vi "Find Candidates.vi"(0 "Target Heading":i16, 1 "Number of Valleys":i16, 2 "START":i16[](array[numeric]), 3 "STOP":i16[](array[numeric]), 5 "Expansion delta":i16) -> (4 "Valley index":i16, 6 "Candidate Direction":i16[](array[numeric]), 7 "Valley Width":i16[](array[numeric]), 8 "Target Bonus":i16[](array[numeric]))   [LabVIEW 2009]
panel:
  out "Target Valley Width":i16
  out "Target Flag":i16
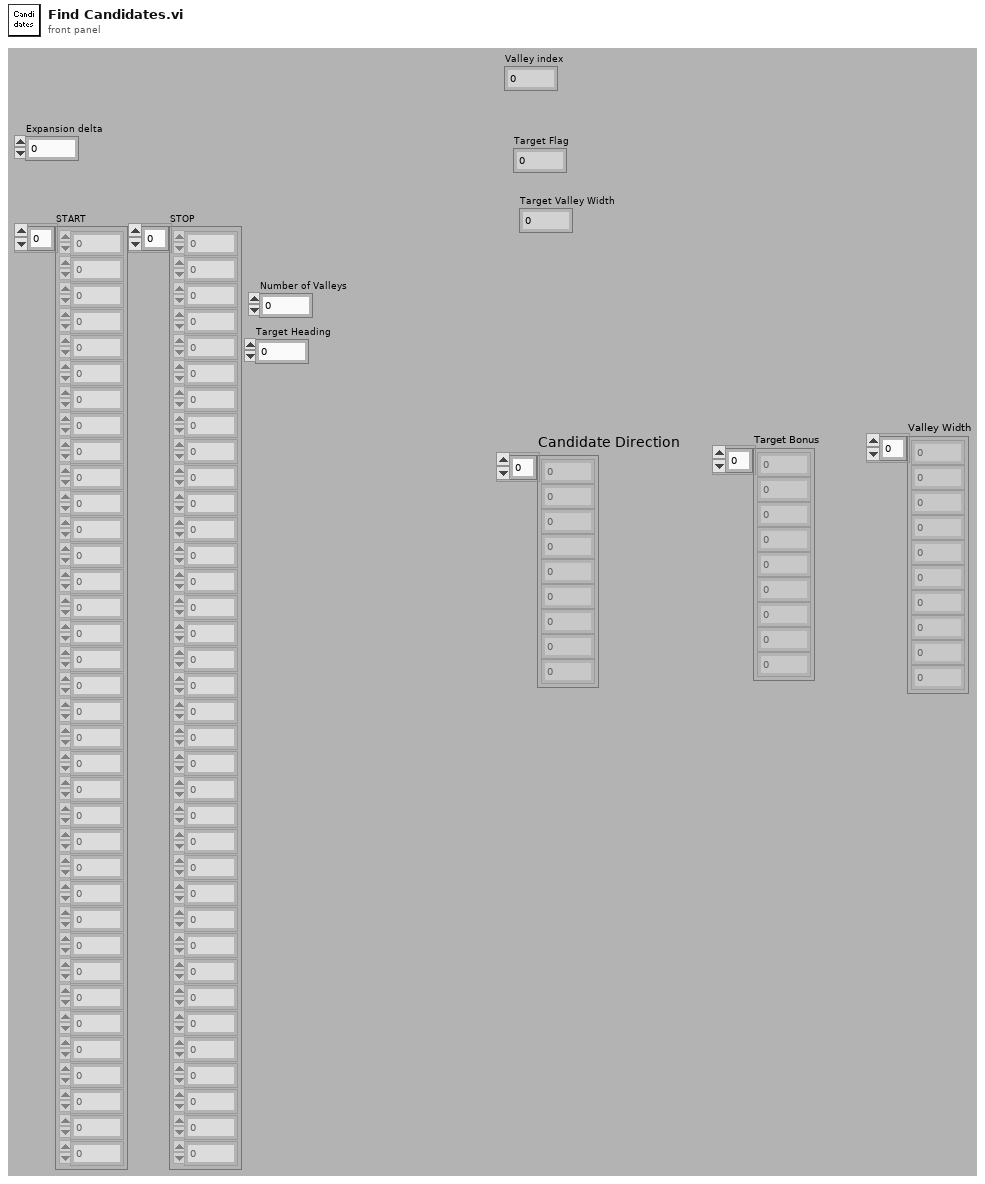
[diagram p1: front panel]
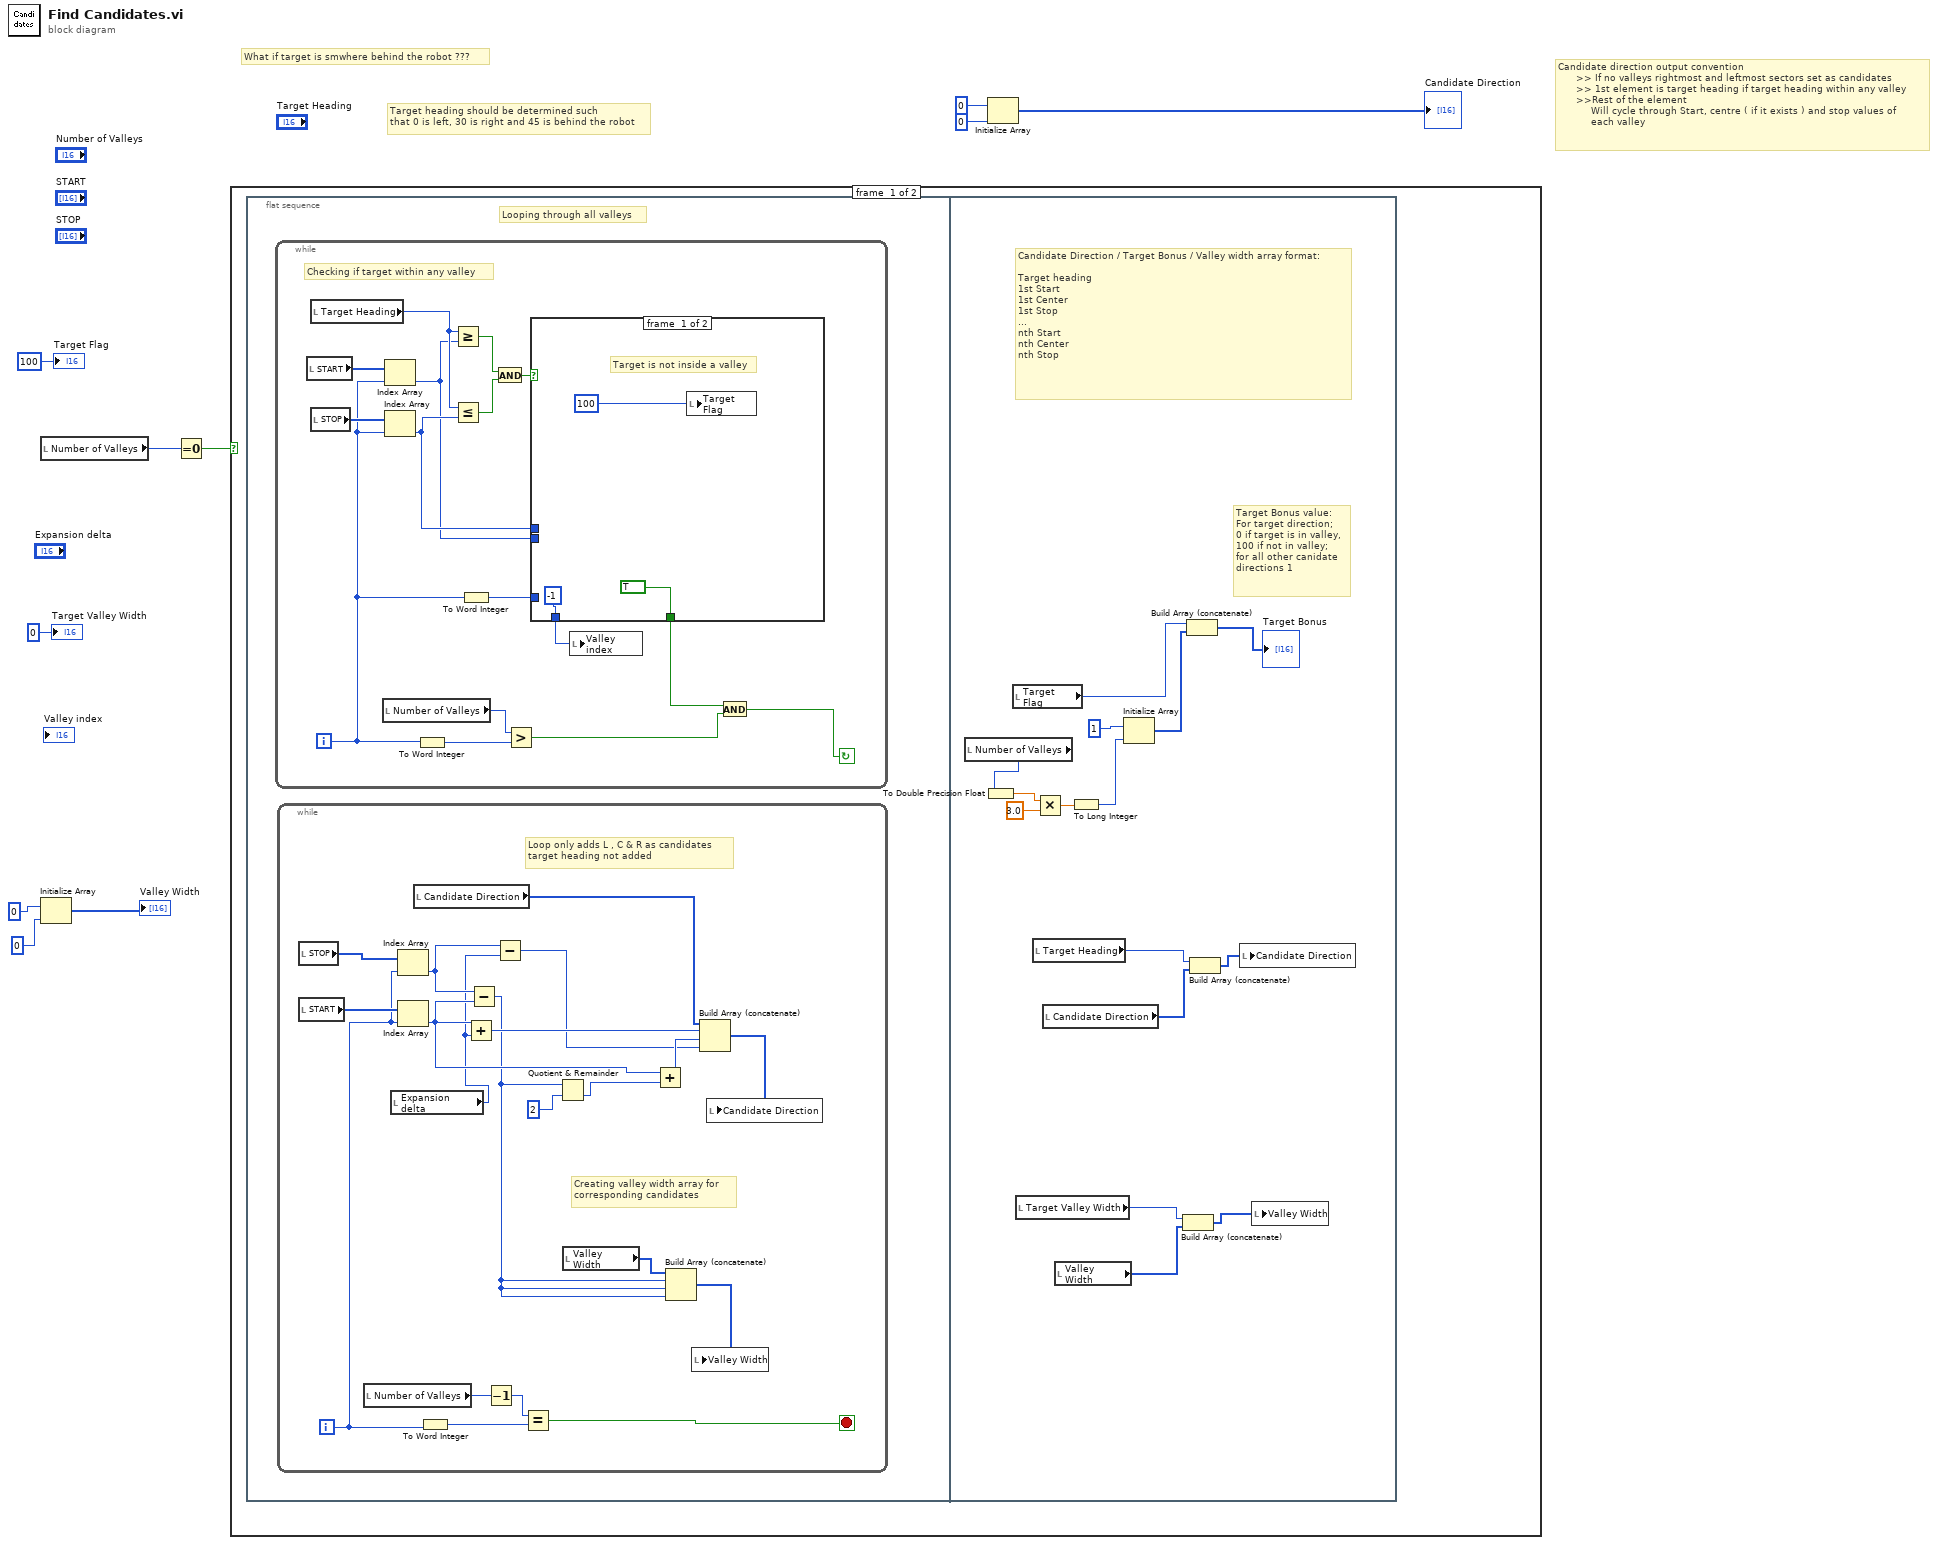
[diagram p0: block diagram]
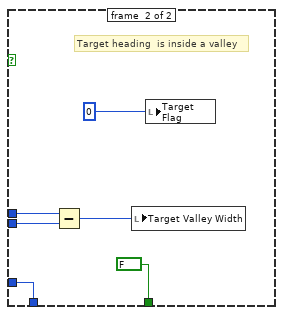
[diagram p2: hidden frame]
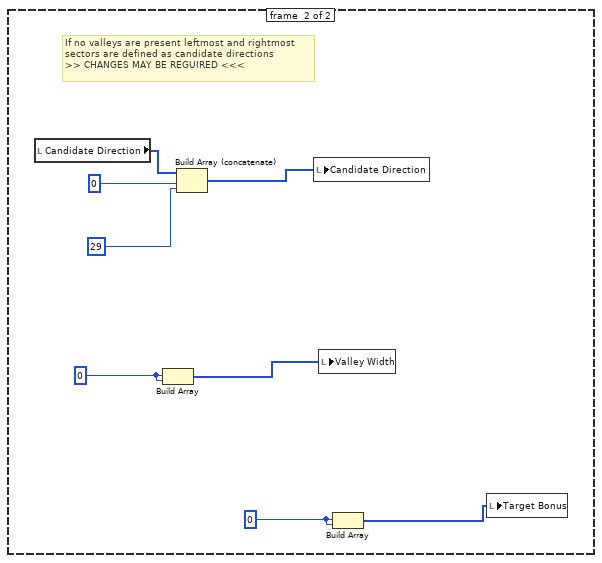
[diagram p3: hidden frame]
diagram:
  # "What if target is smwhere behind the robot ???"
  # "Candidate direction output convention\n      >> If no valleys rightmost and leftmost sectors set as candidates\n      >> 1st element is target heading if target heading within any valley\n      >>Rest of the element\n           Will cycle through Start, centre ( if it exists ) and stop values of\n           each valley"
  # "Target heading should be determined such \nthat 0 is left, 30 is right and 45 is behind the robot"
  n1 = local read "Number of Valleys"() -> (w7:i16)
  n2 = Initialize Array(i16 0 ("element"), 0 ("dimension size")) -> (→"Valley Width":i16[])
  n3 = Equal To 0?(x=w7) -> (x = 0?=w8:bool)
  n4 = case shown="False" w8 {
    frame #0 {
      n5 = flat-sequence {
        frame #0 {
          # "Looping through all valleys"
          n6 = while {
            i -> [w33]
            stop <- w42 continue-if-true
            # "Checking if target within any valley"
            n7 = local read "START"() -> (w45:i16[])
            n8 = local read "Target Heading"() -> (w41:i16)
            n9 = local read "STOP"() -> (w44:i16[])
            n10 = local read "Number of Valleys"() -> (w46:i16)
            n11 = Index Array(array=w45, index=w33) -> (element=w36:i16)
            n12 = Index Array(array=w44, index=w33) -> (element=w37:i16)
            n13 = To Word Integer(number=w33) -> (16bit integer=w34:i16)
            n14 = Greater Or Equal?(x=w41, y=w36) -> (x >= y?=w39:bool)
            n15 = Less Or Equal?(x=w41, y=w37) -> (x <= y?=w38:bool)
            n16 = To Word Integer(number=w33) -> (16bit integer=w31:i16)
            n17 = And(x=w39, y=w38) -> (x .and. y?=w40:bool)
            n18 = Greater?(x=w46, y=w34) -> (0:w43:bool)
            n19 = case shown="False" w40 {
              tunnel: w37 -> [_ w54]
              tunnel: w36 -> [_ w53]
              tunnel: [TRUE FALSE] -> w35
              tunnel: [i16 -1 w50] -> w32
              tunnel: w31 -> [_ w50]
              frame #0 {
                # "Target is not inside a valley"
                n20 = local write "Target Flag"(100 ("Target in Valley ?")) -> ()
              }
              frame #1 {
                # "Target heading  is inside a valley"
                n21 = Subtract(x=w54, y=w53) -> (x-y=w52:i16)
                n22 = local write "Target Valley Width"(w52) -> ()
                n23 = local write "Target Flag"(i16 0 ("Target in Valley")) -> ()
              }
            }
            n24 = local write "Valley index"(w32) -> ()
            n25 = And(x=w35, y=w43) -> (x .and. y?=w42:bool)
          }
          n26 = while {
            i -> [w15]
            stop <- w30 stop-if-true
            # "Creating valley width array for \ncorresponding candidates"
            # "Loop only adds L , C & R as candidates\ntarget heading not added"
            n27 = local read "STOP"() -> (w28:i16[])
            n28 = local read "START"() -> (w29:i16[])
            n29 = local read "Number of Valleys"() -> (w27:i16)
            n30 = local read "Expansion delta"() -> (w16:i16)
            n31 = Index Array(array=w28, index=w15) -> (element=w17:i16)
            n32 = Index Array(array=w29, index=w15) -> (element=w19:i16)
            n33 = local read "Candidate Direction"() -> (w24:i16[])
            n34 = To Word Integer(number=w15) -> (16bit integer=w14:i16)
            n35 = Add(x=w19, y=w16) -> (x+y=w20:i16)
            n36 = Subtract(x=w17, y=w19) -> (x-y=w12:i16)
            n37 = Decrement(x=w27) -> (x-1=w26:i16)
            n38 = Subtract(x=w17, y=w16) -> (x-y=w18:i16)
            n39 = Equal?(x=w26, y=w14) -> (x = y?=w30:bool)
            n40 = Quotient & Remainder(x=w12, y=i16 2) -> (floor(x/y)=w11:i16)  [unwired: 1 out]
            n41 = local read "Valley Width"() -> (w21:i16[])
            n42 = Add(x=w19, y=w11) -> (x+y=w25:i16)
            n43 = Build Array (concatenate)(w21, w12, w12, w12) -> (w22:i16[])
            n44 = local write "Valley Width"(w22) -> ()
            n45 = Build Array (concatenate)(w24, w20, w25, w18) -> (w23:i16[])
            n46 = local write "Candidate Direction"(w23) -> ()
          }
        }
        frame #1 {
          # "Candidate Direction / Target Bonus / Valley width array format:\n\nTarget heading \n1st Start\n1st Center\n1st Stop\n...\nnth Start\nnth Center\nnth Stop"
          # "Target Bonus value:\nFor target direction;\n0 if target is in valley, \n100 if not in valley;\nfor all other canidate \ndirections 1"
          n47 = local read "Number of Valleys"() -> (w58:i16)
          n48 = To Double Precision Float(number=w58) -> (double precision float=w59:dbl)
          n49 = local read "Target Flag"() -> (w66:i16)
          n50 = local read "Target Valley Width"() -> (w61:i16)
          n51 = local read "Target Heading"() -> (w64:i16)
          n52 = Multiply(x=w59, y=3.0) -> (x*y=w57:dbl)
          n53 = local read "Candidate Direction"() -> (w63:i16[])
          n54 = local read "Valley Width"() -> (w62:i16[])
          n55 = To Long Integer(number=w57) -> (32bit integer=w56:i32)
          n56 = Initialize Array(i16 1 ("element"), w56) -> (w68:i16[])
          n57 = Build Array (concatenate)(w61, w62) -> (w60:i16[])
          n58 = Build Array (concatenate)(w66, w68) -> (→"Target Bonus":i16[])
          n59 = Build Array (concatenate)(w64, w63) -> (w65:i16[])
          n60 = local write "Candidate Direction"(w65) -> ()
          n61 = local write "Valley Width"(w60) -> ()
        }
      }
    }
    frame #1 {
      w72 = i16 0
      w71 = i16 0
      # "If no valleys are present leftmost and rightmost\nsectors are defined as candidate directions\n>> CHANGES MAY BE REGUIRED <<<"
      n62 = local read "Candidate Direction"() -> (w78:i16[])
      n63 = Build Array(w71, w71) -> (w74:i16[])
      n64 = Build Array (concatenate)(w78, i16 0, i16 29) -> (w75:i16[])
      n65 = local write "Candidate Direction"(w75) -> ()
      n66 = local write "Valley Width"(w74) -> ()
      n67 = Build Array(w72, w72) -> (w73:i16[])
      n68 = local write "Target Bonus"(w73) -> ()
    }
  }
  n69 = Initialize Array(i16 0 ("element"), 0 ("dimension size")) -> (→"Candidate Direction":i16[])
  "Target Flag" <- i16 100 ("Target in Valley ?")
  "Target Valley Width" <- i16 0 ("Target in Valley ?")
